vi "CloseFPGA.vi"(11 "Reference ID":u64) -> (0 "Error code":i32)   [LabVIEW 2023]
doc: "Closes FPGA reference"
uses:
  <vilib>/FPGAPlugInAG/Dynamic/niLvFpga_Close_Dynamic.vi
  <vilib>/rvi/interface/nirviCloseFPGA/nirviCloseFPGA.xnode
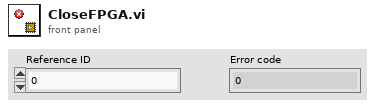
[diagram p1: front panel]
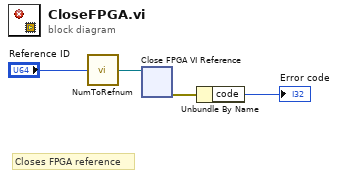
[diagram p0: block diagram]
diagram:
  # "Closes FPGA reference"
  n1 = call "NumToRefnum.vi"("Reference ID"="Reference ID") -> ("Refnum Out"=w4:refnum<k20>)
  n2 = xnode ("Close FPGA VI Reference")("FPGA VI Reference In"=w4) -> ("error out"=w2:errorcluster)  [unwired: 1 in]
  n3 = Unbundle By Name(w2) -> ("code"=→"Error code":i32)
